vi "SetCurrentSettingValueEx.vi"(4 "error in (no error)":errorcluster, 6 "setting value":i32, 7 "axis in":cluster{"keyHandle":u32, "nodeId":u16}={"keyHandle"=0, "nodeId"=1}) -> (0 "error out":errorcluster, 3 "axis out":cluster{"keyHandle":u32, "nodeId":u16}={"keyHandle"=0, "nodeId"=1})   [LabVIEW 2019, in "maxonEPOS.lvlib"]
doc: "<B>SetCurrentSettingValue</B> writes the new current demand value to the device."
uses:
  Examples/maxonEPOS.lvlib
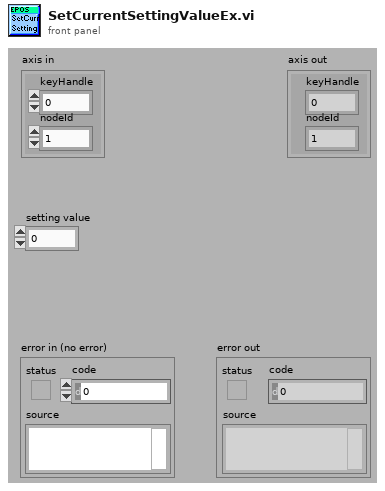
[diagram p1: front panel]
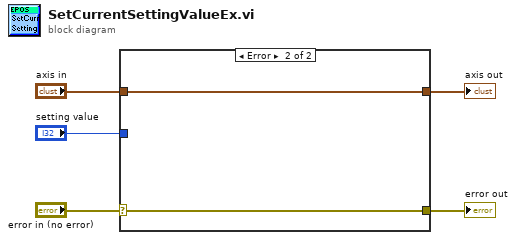
[diagram p0: block diagram]
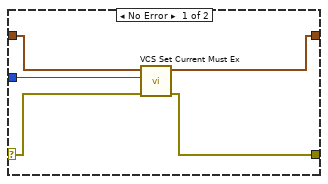
[diagram p2: hidden frame]
diagram:
  n1 = case shown="Error" "error in (no error)" {
    selector: "error in (no error)" -> [w10 w12]
    tunnel: [w9 w12] -> w4
    tunnel: [w8 w11] -> w3
    tunnel: "axis in" -> [w7 w11]
    tunnel: "setting value" -> [w6 _]
    frame No Error {
      n2 = call "VCS Set Current Must Ex.vi"("error in (no error)"=w10, "currentMust"=w6, "axis in"=w7) -> ("error out"=w9:errorcluster, "axis out"=w8:cluster{"keyHandle":u32, "nodeId":u16})  [unwired: 7 in]
    }
    frame Error {
    }
  }
  "error out" <- w4
  "axis out" <- w3
